vi "Initialize Parameters.vi"(8 "error in (no error)":errorcluster, 11 "Data Cluster in":T1) -> (0 "error out":errorcluster, 3 "Data Cluster out":T1)   [LabVIEW 2019, in "Camera.lvlib"]
uses:
  Camera.lvlib
  Module Data--cluster.ctl
  Camera-LVClass/Picam_class/Picam.lvclass
  ROI--cluster.ctl
  picam32_LabView_SDK/PICam_lib/types/PicamGatingMode.ctl
  picam32_LabView_SDK/PICam_lib/types/PicamPulse.ctl
  picam32_LabView_SDK/PICam_lib/PICam.lvlib
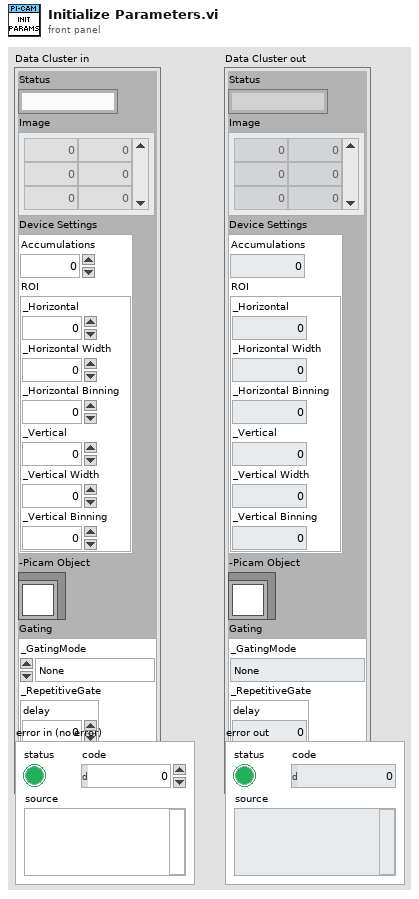
[diagram p1: front panel]
types:
  T1 = typedef "Camera.lvlib/Module Data--cluster.ctl" = cluster{"Status":string, "Image":u16[][], "Device Settings":cluster{"Accumulations":i64, "ROI":T2}, "-Picam Object":refnum<class "Picam.lvclass">, "Gating":cluster{"_GatingMode":T3, "_RepetitiveGate":T4}}
  T2 = typedef "Camera.lvlib/ROI--cluster.ctl" = cluster{"_Horizontal":i32, "_Horizontal Width":i32, "_Horizontal Binning":i32, "_Vertical":i32, "_Vertical Width":i32, "_Vertical Binning":i32}
  T3 = typedef "PICam.lvlib/PicamGatingMode.ctl" = enum16{"None", "Repetitive", "Sequential", "Custom", "Disabled"}
  T4 = typedef "PICam.lvlib/PicamPulse.ctl" = cluster{"delay":dbl, "width":dbl}
  T5 = typedef "Camera.lvlib/Get GatingMode (Reply Payload)--cluster.ctl" = cluster{"PicamGatingMode":T3, "Get GatingMode_error":errorcluster}
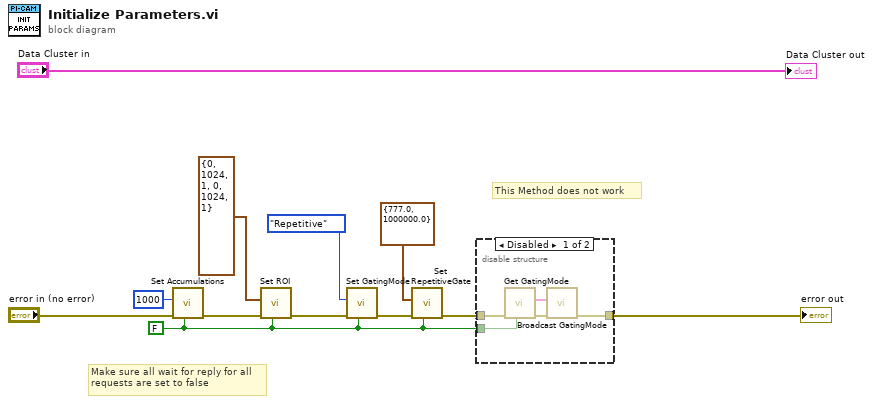
[diagram p0: block diagram]
diagram:
  w1 = FALSE ("wait for reply (T)")
  # "Make sure all wait for reply for all\nrequests are set to false"
  # "This Method does not work"
  n1 = call "Set Accumulations.vi"("wait for reply (T)"=w1, "error in (no error)"="error in (no error)", "Accumulations"=i64 1000) -> ("error out"=w10:errorcluster)  [unwired: 6 in, 2 out]
  n2 = call "Set ROI.vi"("wait for reply (T)"=w1, "error in (no error)"=w10, "ROI"=T2 {"_Horizontal"=0, "_Horizontal Width"=1024, "_Horizontal Binning"=1, "_Vertical"=0, "_Vertical Width"=1024, "_Vertical Binning"=1}) -> ("error out"=w8:errorcluster)  [unwired: 6 in, 2 out]
  n3 = call "Set GatingMode.vi"("wait for reply (T)"=w1, "error in (no error)"=w8, "PicamGatingMode"=PicamGatingMode."Repetitive") -> ("error out"=w5:errorcluster)  [unwired: 6 in, 2 out]
  n4 = call "Set RepetitiveGate.vi"("wait for reply (T)"=w1, "error in (no error)"=w5, "RepetitiveGate"=T4 {"delay"=777.0, "width"=1000000.0}) -> ("error out"=w3:errorcluster)  [unwired: 6 in, 2 out]
  n5 = disable-structure shown="Disabled" {
    disable-tunnel: w3 -> [w17 _]
    disable-tunnel: w1 -> [w15 _]
    disable-tunnel: [w14 _] -> w6
    frame Disabled {
      n6 = call "Get GatingMode.vi"("wait for reply (T)"=w15, "error in (no error)"=w17) -> ("error out"=w16:errorcluster, "Reply Payload"=w13:T5)  [unwired: 7 in, 1 out]
      n7 = call "Broadcast GatingMode.vi"("error in (no error)"=w16, "Reply Payload"=w13) -> ("error out"=w14:errorcluster)  [unwired: 9 in]
    }
    frame Enabled {
    }
  }
  "error out" <- w6
  "Data Cluster out" <- "Data Cluster in"
